vi "Configure Measurement (Phase).vi"(0 "VISA resource name":refnum<visa-resource-name>, 1 "Direction (0: Rising)":i32(ring) items=["Rising", "Falling"], 5 "Measurement Source 1 (1: Channel 1)":i32(ring)=1 caption="Channel (1: Channel 1)" items=["Channel 1"=1, "Channel 2"=2, "Channel 3"=3, "Channel 4"=4, "Function 1"=5, "Function 2"=6, "Function 3"=7, "Function 4"=8, "Memory 1"=9, "Memory 2"=10, "Memory 3"=11, "Memory 4"=12, "Clock"=15, "MTrend"=16, "MSpectrum"=17, "Equalized"=18, "DIG 0"=20, "DIG 1"=21, "DIG 2"=22, "DIG 3"=23, "DIG 4"=24, "DIG 5"=25, "DIG 6"=26, "DIG 7"=27, "DIG 8"=28, "DIG 9"=29, "DIG 10"=30, "DIG 11"=31, "DIG 12"=32, "DIG 13"=33, "DIG 14"=34, "DIG 15"=35], 7 "Measurement Source 2 (2: Channel 2)":i32(ring)=2 caption="Channel (1: Channel 1)" items=["Channel 1"=1, "Channel 2"=2, "Channel 3"=3, "Channel 4"=4, "Function 1"=5, "Function 2"=6, "Function 3"=7, "Function 4"=8, "Memory 1"=9, "Memory 2"=10, "Memory 3"=11, "Memory 4"=12, "Clock"=15, "MTrend"=16, "MSpectrum"=17, "Equalized"=18, "DIG 0"=20, "DIG 1"=21, "DIG 2"=22, "DIG 3"=23, "DIG 4"=24, "DIG 5"=25, "DIG 6"=26, "DIG 7"=27, "DIG 8"=28, "DIG 9"=29, "DIG 10"=30, "DIG 11"=31, "DIG 12"=32, "DIG 13"=33, "DIG 14"=34, "DIG 15"=35], 11 "error in (no error)":errorcluster) -> (4 "VISA resource name out":refnum<visa-resource-name>, 15 "error out":errorcluster)   [LabVIEW 2020, in "Agilent 90000 Series.lvlib"]
doc: "Configures the phase measurement.\n\n<B>Note:</B>\nCalling this VI disables all previously enabled measurements and clears existing measurement results from display."
uses:
  Agilent 90000 Series.lvlib
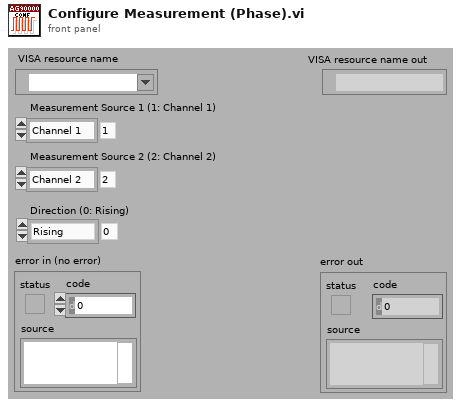
[diagram p1: front panel]
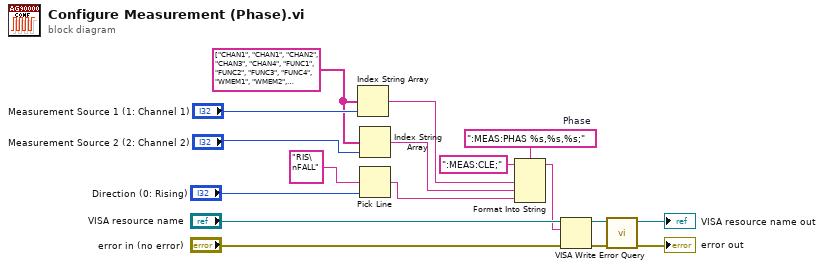
[diagram p0: block diagram]
diagram:
  w1 = string[] ["CHAN1", "CHAN1", "CHAN2", "CHAN3", "CHAN4", "FUNC1", "FUNC2", "FUNC3", "FUNC4", "WMEM1", "WMEM2", "WMEM3", "WMEM4", "AUX", "LINE", "CLOC", "MTR", "MSP", "EQU", "NONE", "DIG0", "DIG1", "DIG2", "DIG3", "DIG4", "DIG5", "DIG6", "DIG7", "DIG8", "DIG9", "DIG10", "DIG11", "DIG12", "DIG13", "DIG14", "DIG15", "", "", "", "", "", "POD1", "POD2", "", "", "", "", "", "", "", "", "BUS1", "BUS2", "BUS3", "BUS4", "", "", "", "", "", "", "DIFF1", "DIFF2", "", "", "", "", "", "", "", "", "COMM3", "COMM4"]
  w10 = ":MEAS:PHAS %s,%s,%s;"  # Phase
  n1 = Index String Array(1:"Measurement Source 1 (1: Channel 1)", 2:w1) -> (0:w9:string)  [unwired: 1 out]
  n2 = Index String Array(1:"Measurement Source 2 (2: Channel 2)", 2:w1) -> (0:w8:string)  [unwired: 1 out]
  n3 = Pick Line(multi-line string="RIS\nFALL", line index="Direction (0: Rising)") -> (output string=w6:string)  [unwired: 1 out]
  n4 = Format Into String(format string=w10, initial string=":MEAS:CLE;", w9, w8, w6) -> (resulting string=w4:string)  [unwired: 1 in, 1 out]
  n5 = VISA Write(VISA resource name="VISA resource name", write buffer=w4, error in (no error)="error in (no error)") -> (VISA resource name out=w13:refnum<visa-resource-name>, error out=w12:errorcluster)  [unwired: 1 out]
  n6 = call "Error Query.vi"("error in (no error)"=w12, "VISA resource name"=w13) -> ("error out"=→"error out":errorcluster, "VISA resource name out"=→"VISA resource name out":refnum<visa-resource-name>)  [unwired: 8 out]
